vi "SequenceSelector_Flush.vi"(1 "Inflow Channel Selector":dbl) -> (0 "Array":u8[][](array[numeric])=[[0, 0, 0, 0, 0, 0, 0, 0, 2, 4, 3, 3, 3, 3], [0, 0, 0, 0, 0, 0, 0, 0, 0, 0, 0, 0, 0, 0], [0, 0, 0, 0, 0, 0, 0, 0, 0, 0, 0, 0, 0, 0], [0, 0, 0, 0, 0, 0, 0, 0, 0, 0, 0, 0, 0, 0], [0, 0, 0, 0, 0, 0, 0, 0, 0, 0, 0, 0, 0, 0], [11, 11, 11, 11, 11, 11, 11, 0, 0, 0, 0, 0, 0, 0], [0, 0, 0, 0, 0, 0, 0, 0, 0, 0, 0, 0, 0, 0], [16, 16, 16, 16, 16, 16, 16, 0, 0, 0, 0, 0, 0, 0], [0, 0, 0, 0, 0, 0, 0, 0, 0, 0, 0, 0, 0, 0], [0, 0, 0, 0, 0, 0, 0, 0, 0, 0, 0, 0, 0, 0], [0, 0, 0, 0, 0, 0, 0, 0, 0, 0, 0, 0, 0, 0], [2, 2, 2, 2, 2, 2, 2, 0, 0, 0, 0, 0, 0, 0], [4, 4, 4, 4, 4, 4, 4, 0, 0, 0, 0, 0, 0, 0], [255, 255, 255, 255, 255, 255, 0, 0, 0, 0, 0, 0, 0, 0], [3, 2, 6, 4, 5, 1, 0, 0, 0, 0, 0, 0, 0, 0], [31, 31, 31, 31, 31, 31, 0, 0, 0, 0, 0, 0, 0, 0], [255, 255, 255, 255, 255, 255, 0, 0, 0, 0, 0, 0, 0, 0]])   [LabVIEW 2016]
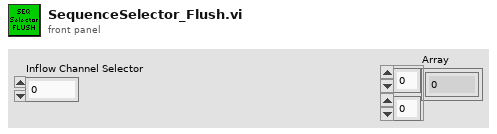
[diagram p1: front panel]
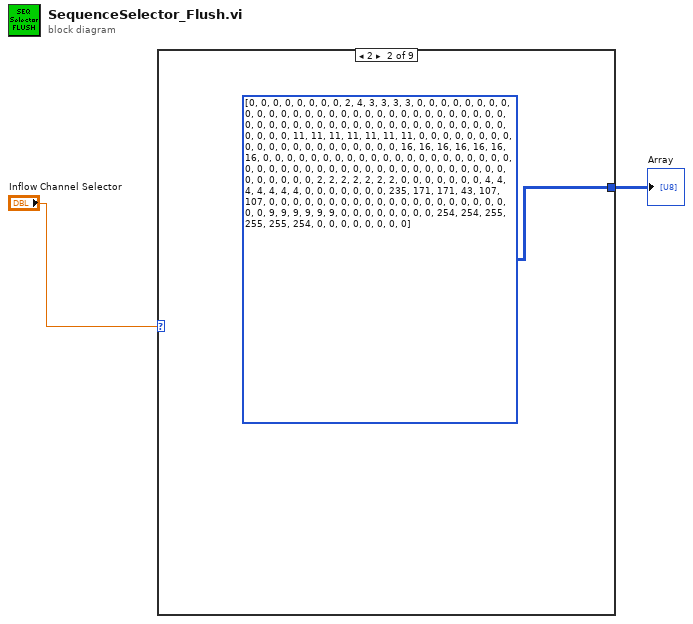
[diagram p0: block diagram]
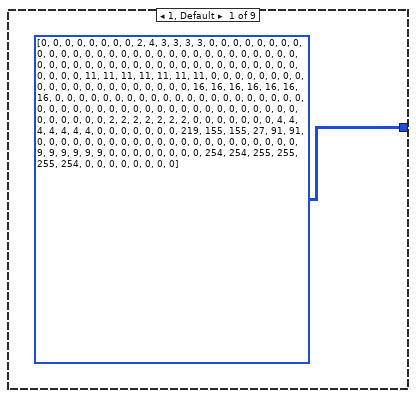
[diagram p2: hidden frame]
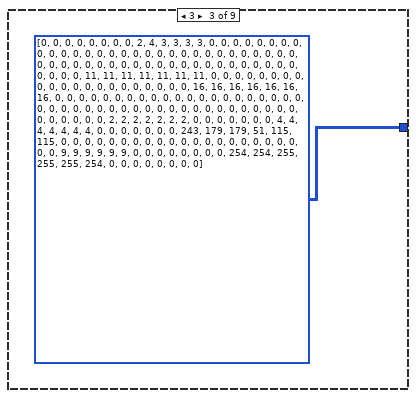
[diagram p3: hidden frame]
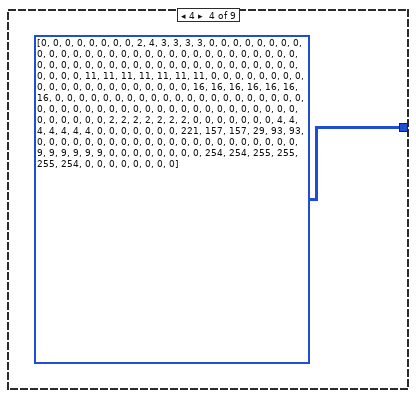
[diagram p4: hidden frame]
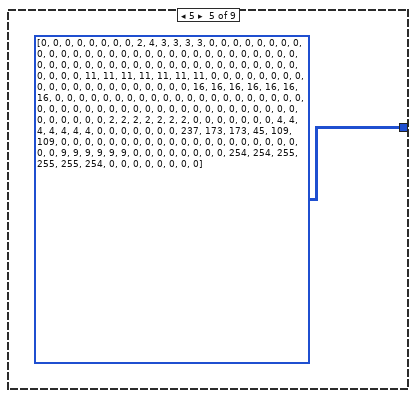
[diagram p5: hidden frame]
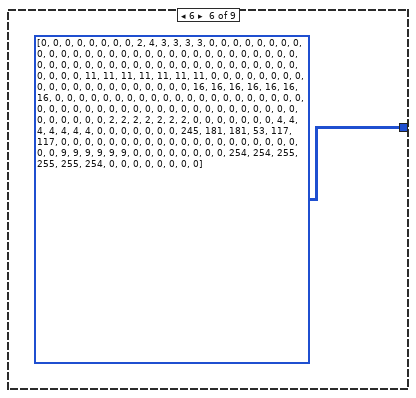
[diagram p6: hidden frame]
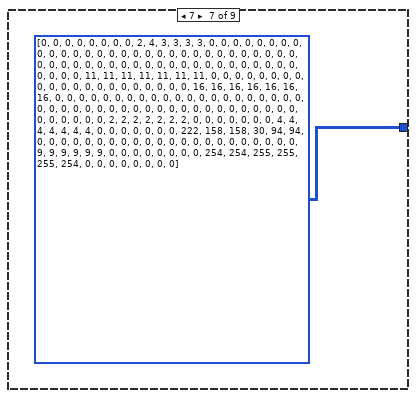
[diagram p7: hidden frame]
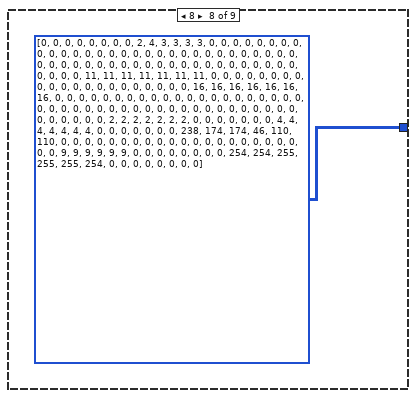
[diagram p8: hidden frame]
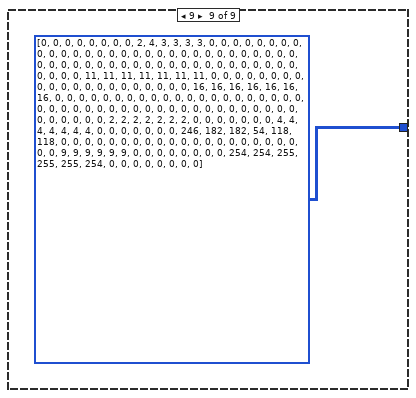
[diagram p9: hidden frame]
diagram:
  n1 = case shown="2" "Inflow Channel Selector" {
    tunnel: [u8[][] [[0, 0, 0, 0, 0, 0, 0, 0, 2, 4, 3, 3, 3, 3], [0, 0, 0, 0, 0, 0, 0, 0, 0, 0, 0, 0, 0, 0], [0, 0, 0, 0, 0, 0, 0, 0, 0, 0, 0, 0, 0, 0], [0, 0, 0, 0, 0, 0, 0, 0, 0, 0, 0, 0, 0, 0], [0, 0, 0, 0, 0, 0, 0, 0, 0, 0, 0, 0, 0, 0], [11, 11, 11, 11, 11, 11, 11, 0, 0, 0, 0, 0, 0, 0], [0, 0, 0, 0, 0, 0, 0, 0, 0, 0, 0, 0, 0, 0], [16, 16, 16, 16, 16, 16, 16, 0, 0, 0, 0, 0, 0, 0], [0, 0, 0, 0, 0, 0, 0, 0, 0, 0, 0, 0, 0, 0], [0, 0, 0, 0, 0, 0, 0, 0, 0, 0, 0, 0, 0, 0], [0, 0, 0, 0, 0, 0, 0, 0, 0, 0, 0, 0, 0, 0], [2, 2, 2, 2, 2, 2, 2, 0, 0, 0, 0, 0, 0, 0], [4, 4, 4, 4, 4, 4, 4, 0, 0, 0, 0, 0, 0, 0], [219, 155, 155, 27, 91, 91, 0, 0, 0, 0, 0, 0, 0, 0], [0, 0, 0, 0, 0, 0, 0, 0, 0, 0, 0, 0, 0, 0], [9, 9, 9, 9, 9, 9, 0, 0, 0, 0, 0, 0, 0, 0], [254, 254, 255, 255, 255, 254, 0, 0, 0, 0, 0, 0, 0, 0]] u8[][] [[0, 0, 0, 0, 0, 0, 0, 0, 2, 4, 3, 3, 3, 3], [0, 0, 0, 0, 0, 0, 0, 0, 0, 0, 0, 0, 0, 0], [0, 0, 0, 0, 0, 0, 0, 0, 0, 0, 0, 0, 0, 0], [0, 0, 0, 0, 0, 0, 0, 0, 0, 0, 0, 0, 0, 0], [0, 0, 0, 0, 0, 0, 0, 0, 0, 0, 0, 0, 0, 0], [11, 11, 11, 11, 11, 11, 11, 0, 0, 0, 0, 0, 0, 0], [0, 0, 0, 0, 0, 0, 0, 0, 0, 0, 0, 0, 0, 0], [16, 16, 16, 16, 16, 16, 16, 0, 0, 0, 0, 0, 0, 0], [0, 0, 0, 0, 0, 0, 0, 0, 0, 0, 0, 0, 0, 0], [0, 0, 0, 0, 0, 0, 0, 0, 0, 0, 0, 0, 0, 0], [0, 0, 0, 0, 0, 0, 0, 0, 0, 0, 0, 0, 0, 0], [2, 2, 2, 2, 2, 2, 2, 0, 0, 0, 0, 0, 0, 0], [4, 4, 4, 4, 4, 4, 4, 0, 0, 0, 0, 0, 0, 0], [235, 171, 171, 43, 107, 107, 0, 0, 0, 0, 0, 0, 0, 0], [0, 0, 0, 0, 0, 0, 0, 0, 0, 0, 0, 0, 0, 0], [9, 9, 9, 9, 9, 9, 0, 0, 0, 0, 0, 0, 0, 0], [254, 254, 255, 255, 255, 254, 0, 0, 0, 0, 0, 0, 0, 0]] u8[][] [[0, 0, 0, 0, 0, 0, 0, 0, 2, 4, 3, 3, 3, 3], [0, 0, 0, 0, 0, 0, 0, 0, 0, 0, 0, 0, 0, 0], [0, 0, 0, 0, 0, 0, 0, 0, 0, 0, 0, 0, 0, 0], [0, 0, 0, 0, 0, 0, 0, 0, 0, 0, 0, 0, 0, 0], [0, 0, 0, 0, 0, 0, 0, 0, 0, 0, 0, 0, 0, 0], [11, 11, 11, 11, 11, 11, 11, 0, 0, 0, 0, 0, 0, 0], [0, 0, 0, 0, 0, 0, 0, 0, 0, 0, 0, 0, 0, 0], [16, 16, 16, 16, 16, 16, 16, 0, 0, 0, 0, 0, 0, 0], [0, 0, 0, 0, 0, 0, 0, 0, 0, 0, 0, 0, 0, 0], [0, 0, 0, 0, 0, 0, 0, 0, 0, 0, 0, 0, 0, 0], [0, 0, 0, 0, 0, 0, 0, 0, 0, 0, 0, 0, 0, 0], [2, 2, 2, 2, 2, 2, 2, 0, 0, 0, 0, 0, 0, 0], [4, 4, 4, 4, 4, 4, 4, 0, 0, 0, 0, 0, 0, 0], [243, 179, 179, 51, 115, 115, 0, 0, 0, 0, 0, 0, 0, 0], [0, 0, 0, 0, 0, 0, 0, 0, 0, 0, 0, 0, 0, 0], [9, 9, 9, 9, 9, 9, 0, 0, 0, 0, 0, 0, 0, 0], [254, 254, 255, 255, 255, 254, 0, 0, 0, 0, 0, 0, 0, 0]] u8[][] [[0, 0, 0, 0, 0, 0, 0, 0, 2, 4, 3, 3, 3, 3], [0, 0, 0, 0, 0, 0, 0, 0, 0, 0, 0, 0, 0, 0], [0, 0, 0, 0, 0, 0, 0, 0, 0, 0, 0, 0, 0, 0], [0, 0, 0, 0, 0, 0, 0, 0, 0, 0, 0, 0, 0, 0], [0, 0, 0, 0, 0, 0, 0, 0, 0, 0, 0, 0, 0, 0], [11, 11, 11, 11, 11, 11, 11, 0, 0, 0, 0, 0, 0, 0], [0, 0, 0, 0, 0, 0, 0, 0, 0, 0, 0, 0, 0, 0], [16, 16, 16, 16, 16, 16, 16, 0, 0, 0, 0, 0, 0, 0], [0, 0, 0, 0, 0, 0, 0, 0, 0, 0, 0, 0, 0, 0], [0, 0, 0, 0, 0, 0, 0, 0, 0, 0, 0, 0, 0, 0], [0, 0, 0, 0, 0, 0, 0, 0, 0, 0, 0, 0, 0, 0], [2, 2, 2, 2, 2, 2, 2, 0, 0, 0, 0, 0, 0, 0], [4, 4, 4, 4, 4, 4, 4, 0, 0, 0, 0, 0, 0, 0], [221, 157, 157, 29, 93, 93, 0, 0, 0, 0, 0, 0, 0, 0], [0, 0, 0, 0, 0, 0, 0, 0, 0, 0, 0, 0, 0, 0], [9, 9, 9, 9, 9, 9, 0, 0, 0, 0, 0, 0, 0, 0], [254, 254, 255, 255, 255, 254, 0, 0, 0, 0, 0, 0, 0, 0]] u8[][] [[0, 0, 0, 0, 0, 0, 0, 0, 2, 4, 3, 3, 3, 3], [0, 0, 0, 0, 0, 0, 0, 0, 0, 0, 0, 0, 0, 0], [0, 0, 0, 0, 0, 0, 0, 0, 0, 0, 0, 0, 0, 0], [0, 0, 0, 0, 0, 0, 0, 0, 0, 0, 0, 0, 0, 0], [0, 0, 0, 0, 0, 0, 0, 0, 0, 0, 0, 0, 0, 0], [11, 11, 11, 11, 11, 11, 11, 0, 0, 0, 0, 0, 0, 0], [0, 0, 0, 0, 0, 0, 0, 0, 0, 0, 0, 0, 0, 0], [16, 16, 16, 16, 16, 16, 16, 0, 0, 0, 0, 0, 0, 0], [0, 0, 0, 0, 0, 0, 0, 0, 0, 0, 0, 0, 0, 0], [0, 0, 0, 0, 0, 0, 0, 0, 0, 0, 0, 0, 0, 0], [0, 0, 0, 0, 0, 0, 0, 0, 0, 0, 0, 0, 0, 0], [2, 2, 2, 2, 2, 2, 2, 0, 0, 0, 0, 0, 0, 0], [4, 4, 4, 4, 4, 4, 4, 0, 0, 0, 0, 0, 0, 0], [237, 173, 173, 45, 109, 109, 0, 0, 0, 0, 0, 0, 0, 0], [0, 0, 0, 0, 0, 0, 0, 0, 0, 0, 0, 0, 0, 0], [9, 9, 9, 9, 9, 9, 0, 0, 0, 0, 0, 0, 0, 0], [254, 254, 255, 255, 255, 254, 0, 0, 0, 0, 0, 0, 0, 0]] u8[][] [[0, 0, 0, 0, 0, 0, 0, 0, 2, 4, 3, 3, 3, 3], [0, 0, 0, 0, 0, 0, 0, 0, 0, 0, 0, 0, 0, 0], [0, 0, 0, 0, 0, 0, 0, 0, 0, 0, 0, 0, 0, 0], [0, 0, 0, 0, 0, 0, 0, 0, 0, 0, 0, 0, 0, 0], [0, 0, 0, 0, 0, 0, 0, 0, 0, 0, 0, 0, 0, 0], [11, 11, 11, 11, 11, 11, 11, 0, 0, 0, 0, 0, 0, 0], [0, 0, 0, 0, 0, 0, 0, 0, 0, 0, 0, 0, 0, 0], [16, 16, 16, 16, 16, 16, 16, 0, 0, 0, 0, 0, 0, 0], [0, 0, 0, 0, 0, 0, 0, 0, 0, 0, 0, 0, 0, 0], [0, 0, 0, 0, 0, 0, 0, 0, 0, 0, 0, 0, 0, 0], [0, 0, 0, 0, 0, 0, 0, 0, 0, 0, 0, 0, 0, 0], [2, 2, 2, 2, 2, 2, 2, 0, 0, 0, 0, 0, 0, 0], [4, 4, 4, 4, 4, 4, 4, 0, 0, 0, 0, 0, 0, 0], [245, 181, 181, 53, 117, 117, 0, 0, 0, 0, 0, 0, 0, 0], [0, 0, 0, 0, 0, 0, 0, 0, 0, 0, 0, 0, 0, 0], [9, 9, 9, 9, 9, 9, 0, 0, 0, 0, 0, 0, 0, 0], [254, 254, 255, 255, 255, 254, 0, 0, 0, 0, 0, 0, 0, 0]] u8[][] [[0, 0, 0, 0, 0, 0, 0, 0, 2, 4, 3, 3, 3, 3], [0, 0, 0, 0, 0, 0, 0, 0, 0, 0, 0, 0, 0, 0], [0, 0, 0, 0, 0, 0, 0, 0, 0, 0, 0, 0, 0, 0], [0, 0, 0, 0, 0, 0, 0, 0, 0, 0, 0, 0, 0, 0], [0, 0, 0, 0, 0, 0, 0, 0, 0, 0, 0, 0, 0, 0], [11, 11, 11, 11, 11, 11, 11, 0, 0, 0, 0, 0, 0, 0], [0, 0, 0, 0, 0, 0, 0, 0, 0, 0, 0, 0, 0, 0], [16, 16, 16, 16, 16, 16, 16, 0, 0, 0, 0, 0, 0, 0], [0, 0, 0, 0, 0, 0, 0, 0, 0, 0, 0, 0, 0, 0], [0, 0, 0, 0, 0, 0, 0, 0, 0, 0, 0, 0, 0, 0], [0, 0, 0, 0, 0, 0, 0, 0, 0, 0, 0, 0, 0, 0], [2, 2, 2, 2, 2, 2, 2, 0, 0, 0, 0, 0, 0, 0], [4, 4, 4, 4, 4, 4, 4, 0, 0, 0, 0, 0, 0, 0], [222, 158, 158, 30, 94, 94, 0, 0, 0, 0, 0, 0, 0, 0], [0, 0, 0, 0, 0, 0, 0, 0, 0, 0, 0, 0, 0, 0], [9, 9, 9, 9, 9, 9, 0, 0, 0, 0, 0, 0, 0, 0], [254, 254, 255, 255, 255, 254, 0, 0, 0, 0, 0, 0, 0, 0]] u8[][] [[0, 0, 0, 0, 0, 0, 0, 0, 2, 4, 3, 3, 3, 3], [0, 0, 0, 0, 0, 0, 0, 0, 0, 0, 0, 0, 0, 0], [0, 0, 0, 0, 0, 0, 0, 0, 0, 0, 0, 0, 0, 0], [0, 0, 0, 0, 0, 0, 0, 0, 0, 0, 0, 0, 0, 0], [0, 0, 0, 0, 0, 0, 0, 0, 0, 0, 0, 0, 0, 0], [11, 11, 11, 11, 11, 11, 11, 0, 0, 0, 0, 0, 0, 0], [0, 0, 0, 0, 0, 0, 0, 0, 0, 0, 0, 0, 0, 0], [16, 16, 16, 16, 16, 16, 16, 0, 0, 0, 0, 0, 0, 0], [0, 0, 0, 0, 0, 0, 0, 0, 0, 0, 0, 0, 0, 0], [0, 0, 0, 0, 0, 0, 0, 0, 0, 0, 0, 0, 0, 0], [0, 0, 0, 0, 0, 0, 0, 0, 0, 0, 0, 0, 0, 0], [2, 2, 2, 2, 2, 2, 2, 0, 0, 0, 0, 0, 0, 0], [4, 4, 4, 4, 4, 4, 4, 0, 0, 0, 0, 0, 0, 0], [238, 174, 174, 46, 110, 110, 0, 0, 0, 0, 0, 0, 0, 0], [0, 0, 0, 0, 0, 0, 0, 0, 0, 0, 0, 0, 0, 0], [9, 9, 9, 9, 9, 9, 0, 0, 0, 0, 0, 0, 0, 0], [254, 254, 255, 255, 255, 254, 0, 0, 0, 0, 0, 0, 0, 0]] u8[][] [[0, 0, 0, 0, 0, 0, 0, 0, 2, 4, 3, 3, 3, 3], [0, 0, 0, 0, 0, 0, 0, 0, 0, 0, 0, 0, 0, 0], [0, 0, 0, 0, 0, 0, 0, 0, 0, 0, 0, 0, 0, 0], [0, 0, 0, 0, 0, 0, 0, 0, 0, 0, 0, 0, 0, 0], [0, 0, 0, 0, 0, 0, 0, 0, 0, 0, 0, 0, 0, 0], [11, 11, 11, 11, 11, 11, 11, 0, 0, 0, 0, 0, 0, 0], [0, 0, 0, 0, 0, 0, 0, 0, 0, 0, 0, 0, 0, 0], [16, 16, 16, 16, 16, 16, 16, 0, 0, 0, 0, 0, 0, 0], [0, 0, 0, 0, 0, 0, 0, 0, 0, 0, 0, 0, 0, 0], [0, 0, 0, 0, 0, 0, 0, 0, 0, 0, 0, 0, 0, 0], [0, 0, 0, 0, 0, 0, 0, 0, 0, 0, 0, 0, 0, 0], [2, 2, 2, 2, 2, 2, 2, 0, 0, 0, 0, 0, 0, 0], [4, 4, 4, 4, 4, 4, 4, 0, 0, 0, 0, 0, 0, 0], [246, 182, 182, 54, 118, 118, 0, 0, 0, 0, 0, 0, 0, 0], [0, 0, 0, 0, 0, 0, 0, 0, 0, 0, 0, 0, 0, 0], [9, 9, 9, 9, 9, 9, 0, 0, 0, 0, 0, 0, 0, 0], [254, 254, 255, 255, 255, 254, 0, 0, 0, 0, 0, 0, 0, 0]]] -> w1
    frame 1, Default {
    }
    frame 2 {
    }
    frame 3 {
    }
    frame 4 {
    }
    frame 5 {
    }
    frame 6 {
    }
    frame 7 {
    }
    frame 8 {
    }
    frame 9 {
    }
  }
  "Array" <- w1
